vi "FPGA_PPG_load_file.vi"(0 "resource_in":refnum<visa-resource-name>, 2 "file_in":path, 5 "error in (no error)":errorcluster) -> (14 "resource_out":refnum<visa-resource-name>, 19 "error out":errorcluster)   [LabVIEW 2014, in "NI-FPGA_PPG_Driver.lvlib"]
doc: "Loads a configuration file to the FPGA target.\n\nContact: Falk Ziegler, eMail: ziegler@physik.uni-greifswald.de"
uses:
  NI-FPGA_PPG_Driver.lvlib
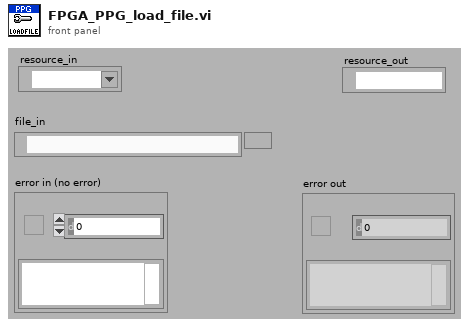
[diagram p1: front panel]
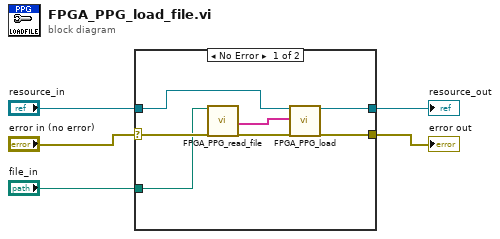
[diagram p0: block diagram]
diagram:
  n1 = case shown="No Error" "error in (no error)" {
    selector: "error in (no error)" -> [w12 w14]
    tunnel: [w7 w14] -> w4
    tunnel: "file_in" -> [w11 _]
    tunnel: "resource_in" -> [w9 w13]
    tunnel: [w8 w13] -> w1
    frame No Error {
      n2 = call "FPGA_PPG_read_file.vi"("file_in"=w11, "error in (no error)"=w12) -> ("cmd_lines"=w6:string[], "error out"=w10:errorcluster)  [unwired: 13 in, 3 out]
      n3 = call "FPGA_PPG_load.vi"("resource_in"=w9, "command_lines"=w6, "error in (no error)"=w10) -> ("resource_out"=w8:refnum<visa-resource-name>, "error out"=w7:errorcluster)  [unwired: 15 in]
    }
    frame Error {
    }
  }
  "error out" <- w4
  "resource_out" <- w1
